vi "Set Button Positions.vi"(4 "Left":i16, 6 "Top":i32, 8 "error in":errorcluster, 10 "label array in":string[](array[string]), 11 "controls[] in":refnum<vi>[](array[refnum])) -> (0 "error out":errorcluster)   [LabVIEW 2018]
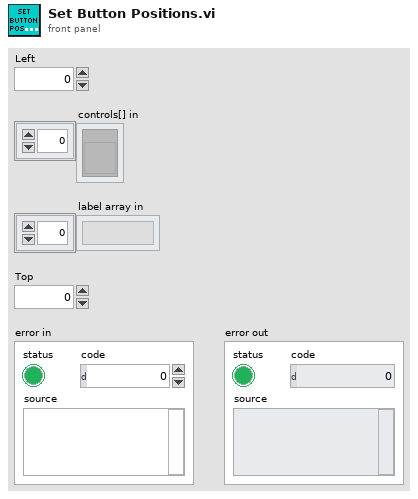
[diagram p1: front panel]
types:
  T1 = typedef "LVRectTypeDef.ctl" = cluster{"Left":i16, "Top":i16, "Right":i16, "Bottom":i16}
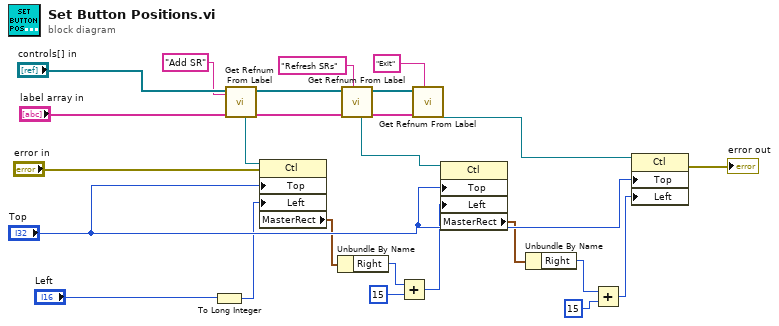
[diagram p0: block diagram]
diagram:
  n1 = To Long Integer(number="Left") -> (32bit integer=w2:i32)
  n2 = call "Get Refnum From Label.vi"("label"="Add SR" ("element"), "label array in"="label array in", "controls[] in"="controls[] in") -> ("label array out"=w21:string[], "controls[] out"=w24:refnum<vi>[], "refnum out"=w17:refnum<vi>)  [unwired: 6 in]
  n3 = property class="Ctl"(reference=w17, error in="error in", "Top"="Top", "Left"=w2) -> ("MasterRect"=w12:T1)  [unwired: 2 out]
  n4 = Unbundle By Name(w12) -> ("Right"=w13:i16)
  n5 = call "Get Refnum From Label.vi"("label"="Refresh SRs" ("element"), "label array in"=w21, "controls[] in"=w24) -> ("label array out"=w22:string[], "controls[] out"=w23:refnum<vi>[], "refnum out"=w20:refnum<vi>)  [unwired: 6 in]
  n6 = Add(x=w13, y=i16 15) -> (x+y=w11:i16)
  n7 = call "Get Refnum From Label.vi"("label"="Exit" ("element"), "label array in"=w22, "controls[] in"=w23) -> ("refnum out"=w19:refnum<vi>)  [unwired: 6 in, 2 out]
  n8 = property class="Ctl"(reference=w20, "Top"="Top", "Left"=w11) -> ("MasterRect"=w6:T1)  [unwired: 1 in, 2 out]
  n9 = Unbundle By Name(w6) -> ("Right"=w5:i16)
  n10 = Add(x=w5, y=i16 15) -> (x+y=w4:i16)
  n11 = property class="Ctl"(reference=w19, "Top"="Top", "Left"=w4) -> (error out=→"error out":errorcluster)  [unwired: 1 in, 1 out]
